vi "Main.vi"(10 "DAQ Type":enum16{"Hardware", "Simulation"}(ring), 11 "Module Admin":refnum<class "Delacor_lib_QMH_Module Admin.lvclass">) -> ()   [LabVIEW 2016, in "CAN.lvlib"]
doc: "This template is based off of the Queued Message Handler design pattern and the Queued Message Handler project template that ships with LabVIEW.\n\nThe main difference is that the queue is private to this module and communication between modules is performed via Broadcast and Request events.\n\nRequest events are wrapped in public API methods and are handled in the Event Handling Loop (EHL) of this VI. Any module can register for Broadcast events sent by this module. The EHL generates messages based on user interface actions.\n\nThe Message Handling Loop (MHL) processes messages generated by the EHL, or by other messages. The messages are string values, so new messages can be added easily to the Message Cases case structure in the MHL. Each message cluster can also provide an optional value for Message Data, which is a variant that can be converted to whatever message-specific data is required.\n_____\nBased on DQMH Project Template 6.1.0.94."
uses:
  CAN.lvlib
  <vilib>/Delacor/Delacor QMH/Libraries/Module Admin_class/Delacor_lib_QMH_Module Admin.lvclass
  Class/Abstract/Abstract.lvclass
  Class/PXI 8513/PXI 8513.lvclass
  D:/common_ATE/Libraries/CAN/Class/Abstract/Abstract.lvclass
  Module Data--cluster.ctl
  <vilib>/Delacor/Delacor QMH/Libraries/Message Queue_class/Delacor_lib_QMH_Message Queue.lvclass/Delacor_lib_QMH_Message Queue.ctl
  Stop Argument--cluster.ctl
  <vilib>/Delacor/Delacor QMH/Libraries/Module Admin_class/Delacor_lib_QMH_Module Admin.lvclass/Delacor_lib_QMH_Module Admin.ctl
  REQ Initialize Hardware Argument--cluster.ctl
  REQ Initialize Hardware (Reply Payload)--cluster.ctl
  REQ Setup Argument--cluster.ctl
  REQ Get Channel Data Argument--cluster.ctl
  REQ CAN Data Argument--cluster.ctl
  REQ Close Ref Argument--cluster.ctl
  <vilib>/Utility/miscctls.llb/LVPointTypeDef.ctl
  <vilib>/Delacor/Delacor QMH/Libraries/Message Queue_class/Delacor_lib_QMH_Enqueue Message (Single).vi
  <vilib>/Delacor/Delacor QMH/Libraries/Module Admin_class/Delacor_lib_QMH_Get External Launch.vi
  <vilib>/Utility/error.llb/Error Cluster From Error Code.vi
  <vilib>/ErrorRing/Error Ring.xnode
  REQ Create CAN Database Argument--cluster.ctl
  <vilib>/Delacor/Delacor QMH/Libraries/Message Queue_class/Delacor_lib_QMH_Message Queue.lvclass
panel:
  out "Session Setting":T1
  out "interface":refnum<k21>
  out "signal list":refnum<k21>[](array[refnum])
  out "Abstract.lvclass":refnum<class "Abstract.lvclass">
  in  "CAN Read?":bool
  out "error out":errorcluster
  out "Status":string
  in  "Simulate MHL Error":bool
  in  "Simulate EHL Error":bool
  # "Other QMH Modules communicate with this Module via its Public API (wrappers for its Request Events).\n\nThis Module communicates with other Modules via its Broadcast Events.\nAny module that wants to get these messages, just registers for this module's Broadcast events."
  # "This template is for the Delacor Modified Queued Message Handler design pattern.\n\nSee the block diagram for more information on how to use this template."
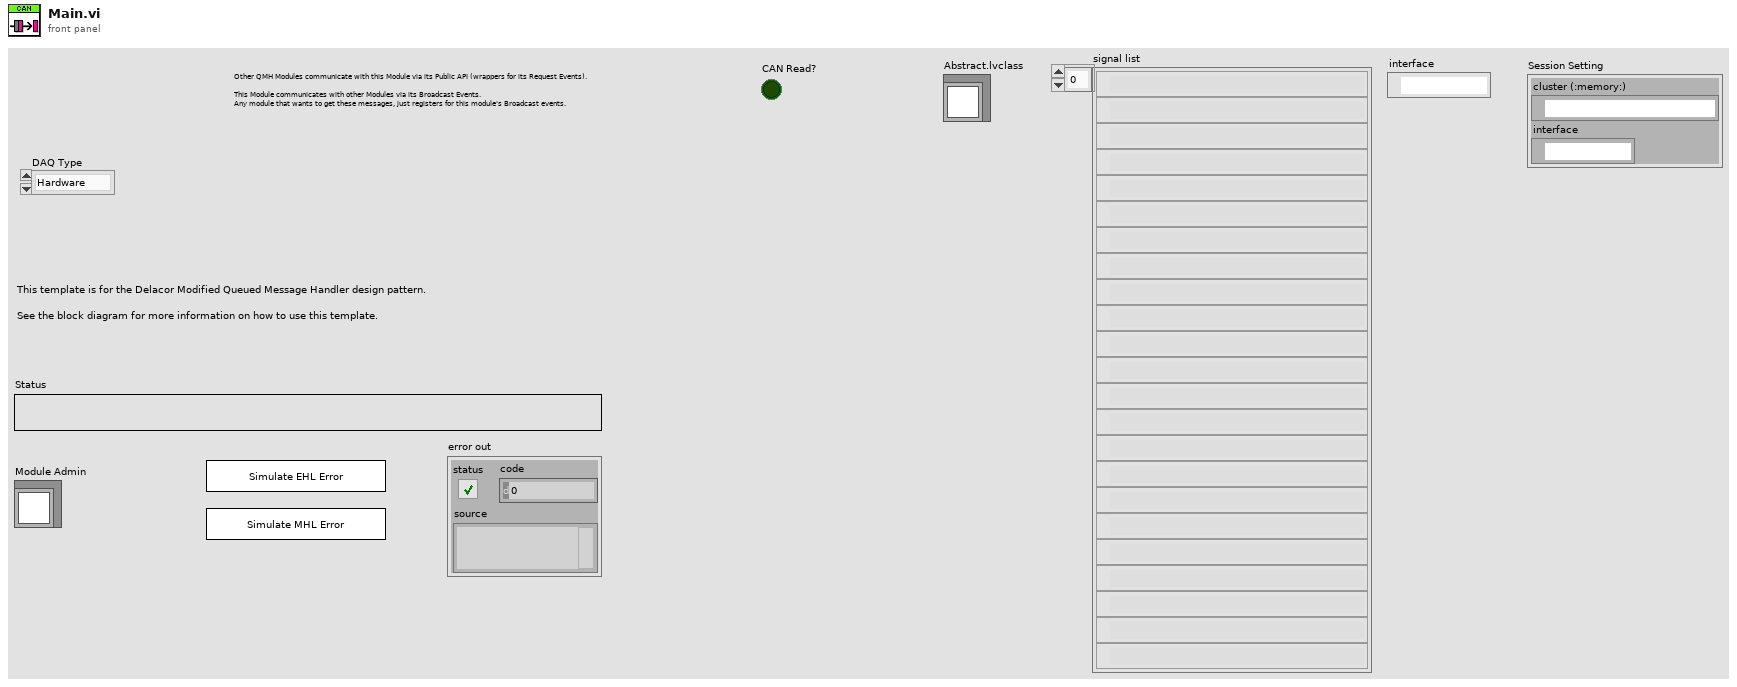
[diagram p1: front panel]
types:
  T1 = cluster{"cluster (:memory:)":refnum<k21>, "interface":refnum<k21>}
  T2 = typedef "CAN.lvlib/Request Events--cluster.ctl" = cluster{"Stop Module":refnum<user-event>, "Show Panel":refnum<user-event>, "Hide Panel":refnum<user-event>, "Get Module Execution Status":refnum<user-event>, "Show Diagram":refnum<user-event>, "REQ Initialize Hardware":refnum<user-event>, "REQ Setup":refnum<user-event>, "REQ Get Channel Data":refnum<user-event>, "REQ CAN Data":refnum<user-event>, "REQ Close Ref":refnum<user-event>, "REQ Create CAN Database":refnum<user-event>}
  T3 = typedef "CAN.lvlib/Module Data--cluster.ctl" = cluster{"Status":string, "Abstract.lvclass":refnum<class "Abstract.lvclass">, "Session Setting":cluster{"cluster (:memory:)":refnum<k21>, "interface":refnum<k21>}, "signal list":refnum<k21>[], "interface":refnum<k21>}
  T4 = enum32{"invalid lock state", "Not Locked", "Locked (No Password)", "Password-protected"}
  T5 = typedef "CAN.lvlib/Stop Argument--cluster.ctl" = cluster{"Origin":string, "Exit via Stop Module Req?":bool, "Wait for Module to stop?":bool}
  T6 = typedef "CAN.lvlib/REQ Initialize Hardware Argument--cluster.ctl" = cluster{"Session Setting":cluster{"cluster (:memory:)":refnum<k21>, "interface":refnum<k21>}, "Connection Ref":variant, "Wait Notifier":refnum<notifier>, "wait for reply":bool}
  T7 = typedef "CAN.lvlib/REQ Setup Argument--cluster.ctl" = cluster{"Setup Setting":cluster{"Interface:64bit Baud Rate":u64, "Interface:CAN:Termination":u32, "Interface:Echo Transmit?":bool}}
  T8 = typedef "CAN.lvlib/REQ Get Channel Data Argument--cluster.ctl" = cluster{"Boolean":bool, "signal list":refnum<k21>[], "interface":refnum<k21>}
  T9 = typedef "CAN.lvlib/REQ CAN Data Argument--cluster.ctl" = cluster{"CAN Read?":bool}
  T10 = typedef "CAN.lvlib/REQ Close Ref Argument--cluster.ctl" = cluster{"Boolean":bool}
  T11 = typedef "CAN.lvlib/REQ Create CAN Database Argument--cluster.ctl" = cluster{"Database Configuration":cluster{"Interface":refnum<k21>, "CAN Cluster":cluster{"Baud Rate":u32, "Comment":string, "Name":string}, "CAN Frame":cluster{"Frame name":string, "Identifier":u32, "Payload Length":u32, "Timing Type":u32, "Transmit Time":dbl, "Extended Identifier?":bool, "Comment":string}, "Signal Cluster":cluster{"Signal name":string, "Scaling Factor":dbl, "Scaling Offset":dbl, "Maximum Value":dbl, "Minimum Value":dbl, "Default Value":dbl, "Unit":string, "Start Bit":u32, "Number of Bits":u32, "Data Type":u32, "Byte Order":u32, "Comment":string}, "Session Type (All Single Point)":enum32{"Signal Input", "Signal Output", "Frame Input", "Frame Output"}}}
  T12 = typedef "LVPointTypeDef.ctl" = cluster{"Horizontal":i16, "Vertical":i16}
  T13 = enum32{"Invalid", "Standard", "Closed", "Hidden", "Minimized", "Maximized"}
  T14 = typedef "CAN.lvlib/REQ Initialize Hardware (Reply Payload)--cluster.ctl" = cluster{"Connect?":bool, "error":errorcluster}
  T15 = cluster{"Interface:64bit Baud Rate":u64, "Interface:CAN:Termination":u32, "Interface:Echo Transmit?":bool}
  T16 = cluster{"Interface":refnum<k21>, "CAN Cluster":cluster{"Baud Rate":u32, "Comment":string, "Name":string}, "CAN Frame":cluster{"Frame name":string, "Identifier":u32, "Payload Length":u32, "Timing Type":u32, "Transmit Time":dbl, "Extended Identifier?":bool, "Comment":string}, "Signal Cluster":cluster{"Signal name":string, "Scaling Factor":dbl, "Scaling Offset":dbl, "Maximum Value":dbl, "Minimum Value":dbl, "Default Value":dbl, "Unit":string, "Start Bit":u32, "Number of Bits":u32, "Data Type":u32, "Byte Order":u32, "Comment":string}, "Session Type (All Single Point)":enum32{"Signal Input", "Signal Output", "Frame Input", "Frame Output"}}
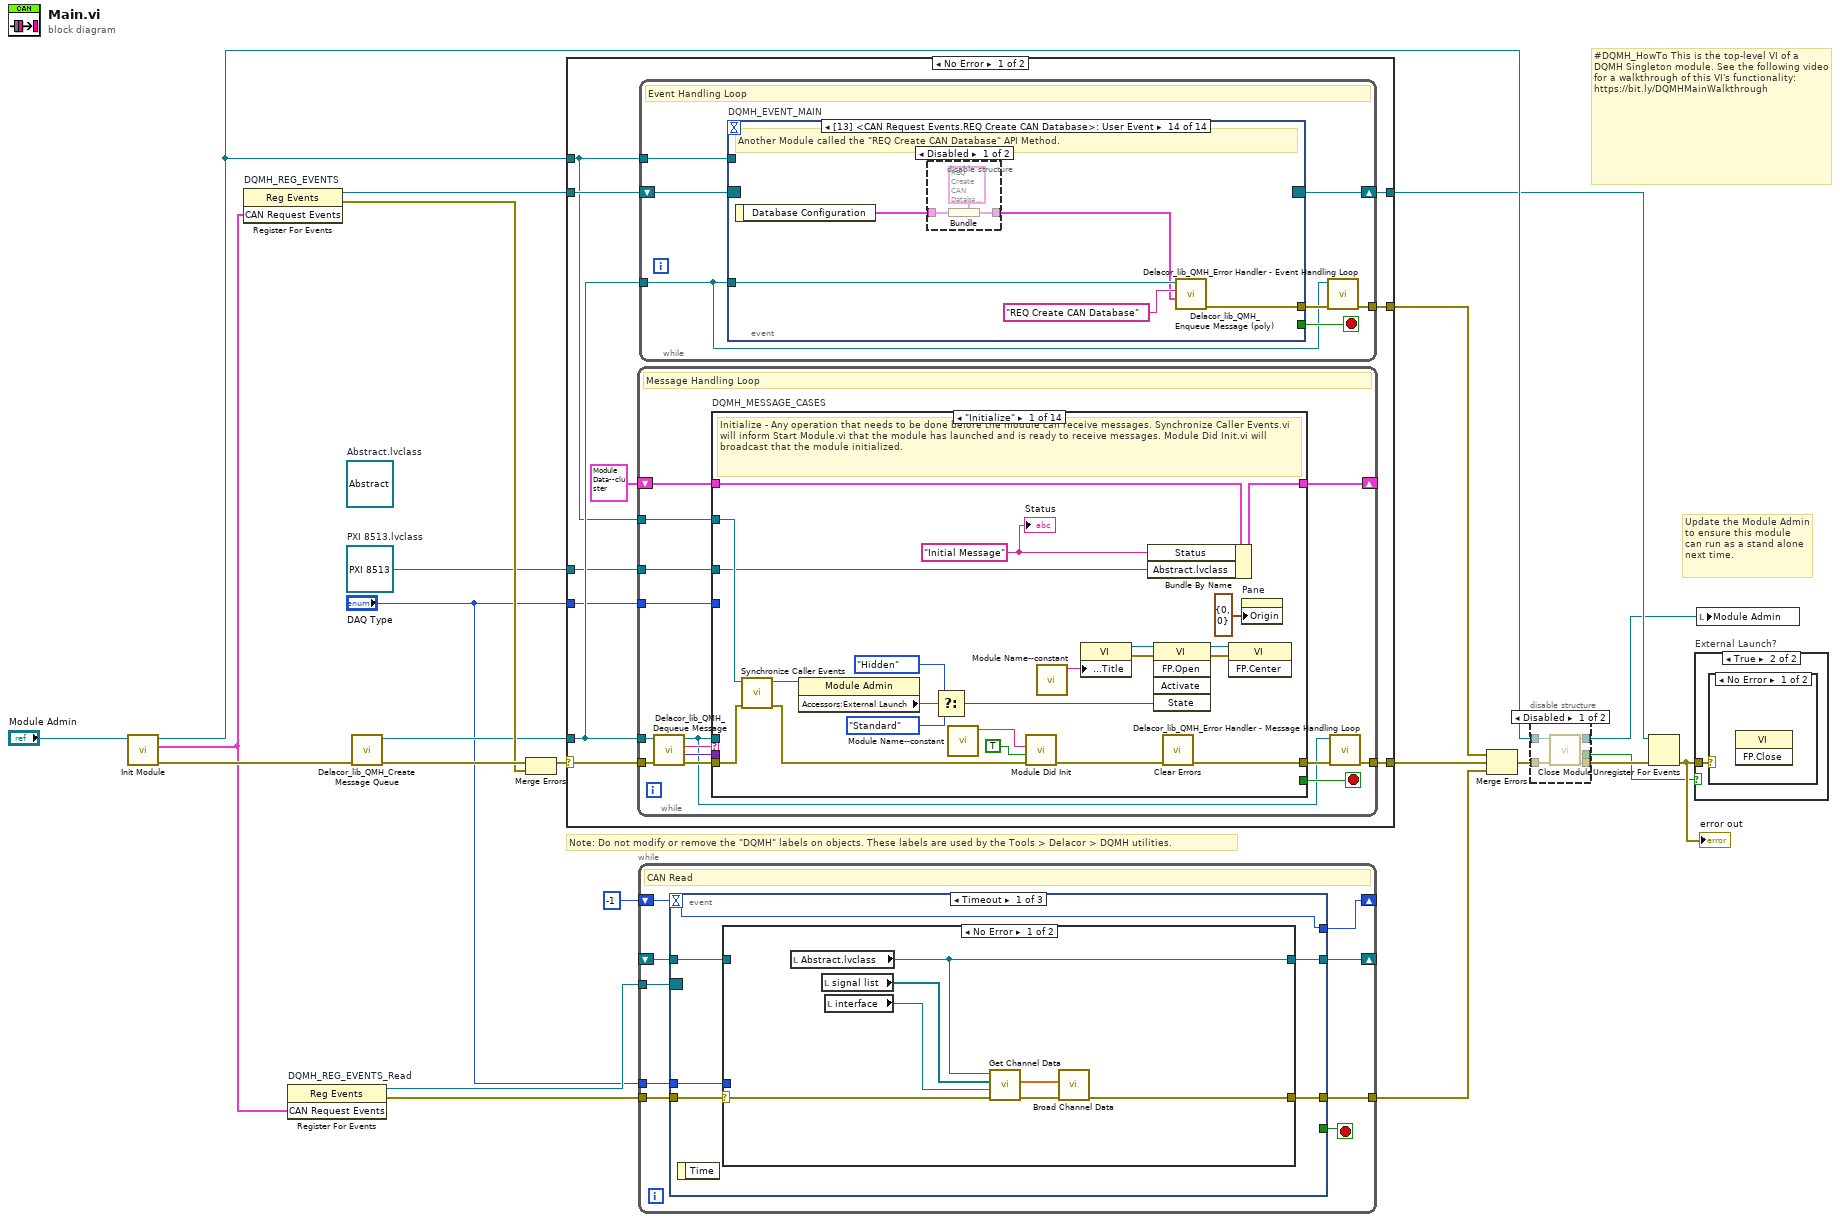
[diagram p0: block diagram]
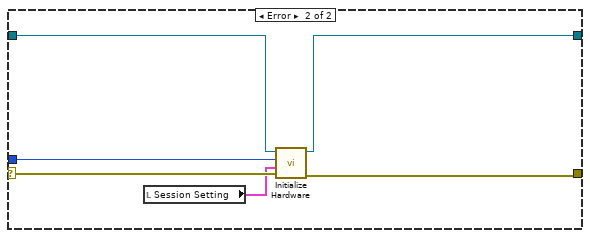
[diagram p3: hidden frame]
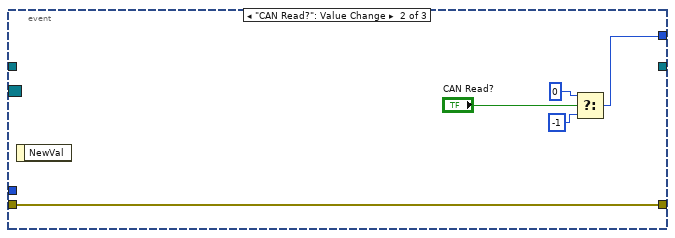
[diagram p4: hidden frame]
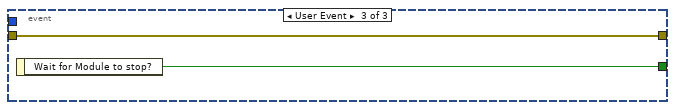
[diagram p5: hidden frame]
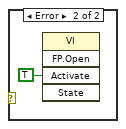
[diagram p7: hidden frame]
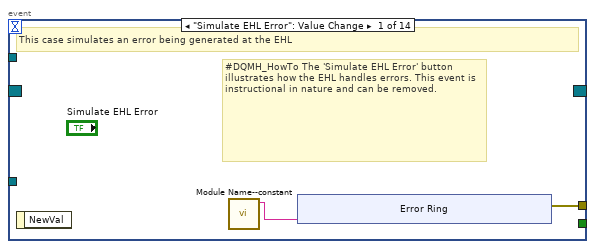
[diagram p8: hidden frame]
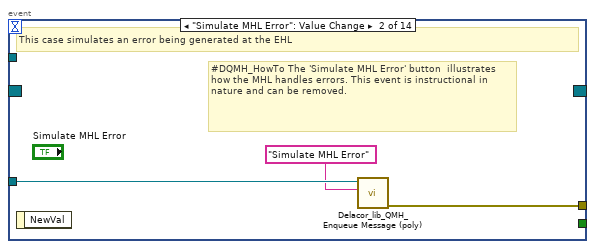
[diagram p9: hidden frame]
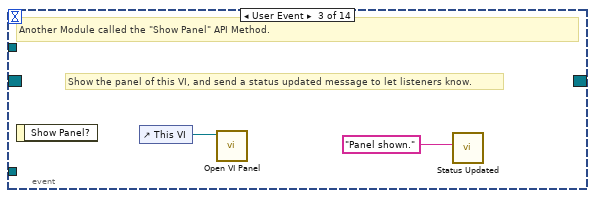
[diagram p10: hidden frame]
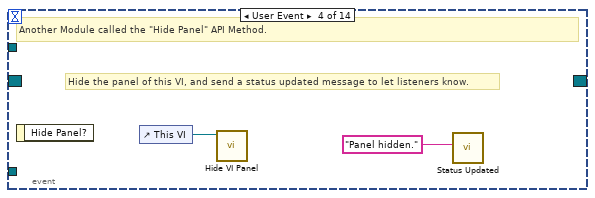
[diagram p11: hidden frame]
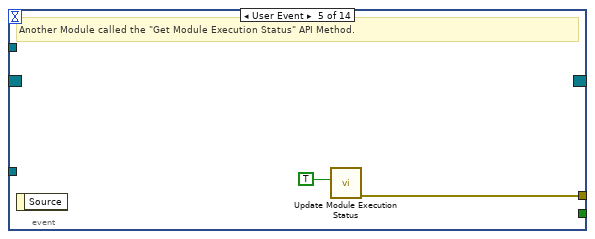
[diagram p12: hidden frame]
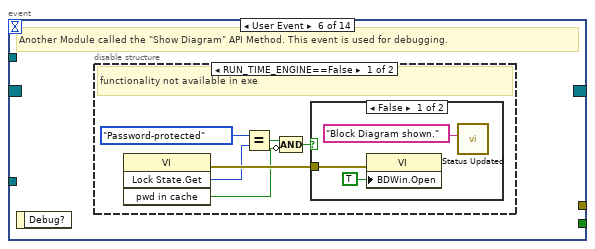
[diagram p13: hidden frame]
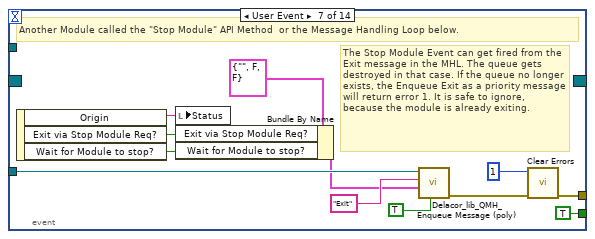
[diagram p16: hidden frame]
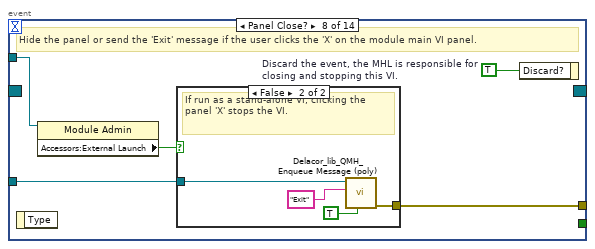
[diagram p17: hidden frame]
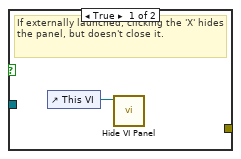
[diagram p18: hidden frame]
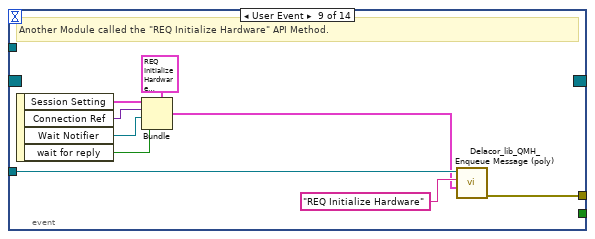
[diagram p19: hidden frame]
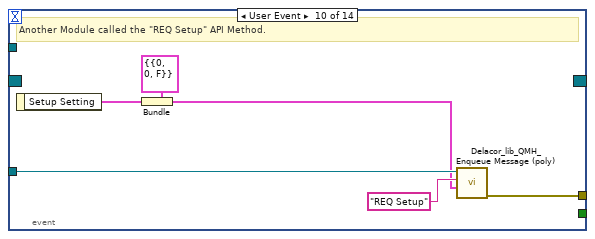
[diagram p20: hidden frame]
diagram:
  w7 = refnum<class "PXI 8513.lvclass"> refnum  # PXI 8513.lvclass
  (unwired) refnum<class "Abstract.lvclass"> refnum  # Abstract.lvclass
  # "#DQMH_HowTo This is the top-level VI of a DQMH Singleton module. See the following video for a walkthrough of this VI's functionality: https://bit.ly/DQMHMainWalkthrough"
  # "Note: Do not modify or remove the \"DQMH\" labels on objects. These labels are used by the Tools > Delacor > DQMH utilities."
  # "Update the Module Admin to ensure this module can run as a stand alone next time."
  n1 = call "Init Module.vi"("Singleton Module Admin in"="Module Admin") -> ("error out"=w22:errorcluster, "CAN Request Events"=w6:T2, "Singleton Module Admin out"=w14:refnum<class "Delacor_lib_QMH_Module Admin.lvclass">)  [unwired: 8 in]
  n2 = register-events "DQMH_REG_EVENTS"(w6) -> (reference out=w12:refnum<event-registration>, error out=w15:errorcluster)  [unwired: 2 in]
  n3 = register-events "DQMH_REG_EVENTS_Read"(w6) -> (reference out=w5:refnum<event-registration>, error out=w4:errorcluster)  [unwired: 2 in]
  n4 = call <vilib>:"Delacor_lib_QMH_Create Message Queue.vi"("error in"=w22) -> ("error out"=w17:errorcluster, "Message Queue"=w11:refnum<class "Delacor_lib_QMH_Message Queue.lvclass">)  [unwired: 9 in]
  n5 = Merge Errors(w17, w15) -> (w16:errorcluster)
  n6 = case shown="No Error" w16 {
    selector: w16 -> [w31 w320]
    tunnel: [w33 w319] -> w23
    tunnel: [w30 w325] -> w13
    tunnel: w12 -> [w28 w325]
    tunnel: w11 -> [w27 w318]
    tunnel: [w32 _] -> w20
    tunnel: w14 -> [w26 w321]
    tunnel: w7 -> [w25 _]
    tunnel: "DAQ Type" -> [w24 _]
    frame No Error {
      n7 = while {
        tunnel: w27 -> [w137]
        shift-right: [w141] -> _
        shift-left: T3 {"Status"="", "Abstract.lvclass"=refnum, "Session Setting"={"cluster (:memory:)"=":memory:", "interface"=""}, "signal list"=[], "interface"=""} ("Data Cluster") -> [w142]
        tunnel: w31 -> [w145]
        tunnel: [w143] -> w33
        tunnel: w26 -> [w135]
        tunnel: w25 -> [w134]
        tunnel: w24 -> [w133]
        stop <- w140 stop-if-true
        # "Message Handling Loop"
        n8 = call-dynamic "Delacor_lib_QMH_Dequeue Message.vi"("error in"=w145, "Message Queue in"=w137) -> ("error out"=w144:errorcluster, "Message Data"=w138:variant, "Message"=w139:string, "Message Queue out"=w136:refnum<class "Delacor_lib_QMH_Message Queue.lvclass">)  [unwired: 6 in]
        n9 = case "DQMH_MESSAGE_CASES" shown="\"Initialize\"" w139 {
          selector: w139 -> [_ _ _ _ _ _ _ _ _ _ _ _ _ w305]
          tunnel: w136 -> [_ _ _ _ _ _ _ _ _ _ _ w271 w293 _]
          tunnel: w144 -> [w166 w170 w189 w202 w211 w223 w229 w239 w254 w256 w261 w278 w299 w307]
          tunnel: [w147 w170 w171 w197 w209 w217 w224 w234 w253 w256 w260 w274 w296 w308] -> w146
          tunnel: w142 -> [w155 w169 w173 w195 w210 w216 w225 w233 w252 w255 w258 w273 w292 w306]
          tunnel: [w154 w169 w180 w193 w205 w216 w225 w231 w252 w255 w258 w273 w292 w306] -> w141
          tunnel: [_ _ _ _ _ _ _ _ _ _ _ _ w291 _] -> w140
          tunnel: w138 -> [_ _ w188 w201 w208 w222 w228 w238 _ _ _ w272 w290 _]
          tunnel: w135 -> [w156 _ _ _ _ _ _ _ _ _ _ w270 w285 _]
          tunnel: w134 -> [w148 _ _ _ _ _ _ _ _ _ _ _ _ _]
          tunnel: w133 -> [_ _ w176 _ _ _ _ _ _ _ _ _ _ _]
          frame "Initialize" {
            w150 = "Initial Message" ("Initial Message")
            # "Initialize - Any operation that needs to be done before the module can receive messages. Synchronize Caller Events.vi will inform Start Module.vi that the module has launched and is ready to receive messages. Module Did Init.vi will broadcast that the module initialized."
            n10 = call "Synchronize Caller Events.vi"("error in (no error)"=w166, "Singleton Module Admin in"=w156) -> ("error out"=w165:errorcluster, "Singleton Module Admin out"=w151:refnum<class "Delacor_lib_QMH_Module Admin.lvclass">)  [unwired: 8 in]
            n11 = property class="Module Admin"(reference=w151) -> ("Accessors:External Launch"=w160:bool)  [unwired: 1 in, 2 out]
            n12 = Select(t=T13."Hidden" ("State"), s=w160, f=T13."Standard" ("State")) -> (s? t:f=w157:T13)
            n13 = call "Module Name--constant.vi"() -> ("Module Name"=w152:string)  [unwired: 11 in]
            n14 = call "Module Did Init.vi"("error in (no error)"=w165, "Initialized?"=TRUE, "Origin"=w152) -> ("error out"=w164:errorcluster)  [unwired: 8 in]
            n15 = call "Module Name--constant.vi"() -> ("Module Name"=w163:string)  [unwired: 11 in]
            n16 = property class="VI"("Front Panel.Title"=w163) -> (reference out=w162:refnum<vi>, error out=w168:errorcluster)  [unwired: 2 in]
            n17 = Bundle By Name(cluster=w155, "Status"=w150, "Abstract.lvclass"=w148) -> (w154:T3)
            n18 = invoke class="VI" method="FP.Open"(reference=w162, error in=w168, "State"=w157) -> (reference out=w161:refnum<vi>, error out=w167:errorcluster)  [unwired: 2 in, 3 out]
            n19 = call <vilib>:"Clear Errors.vi"("error in (no error)"=w164) -> ("error out"=w147:errorcluster)  [unwired: 5 in, 1 out]
            n20 = invoke class="VI" method="FP.Center"(reference=w161, error in=w167) -> ()  [unwired: 1 in, 3 out]
            n21 = property on="Pane" class="Pane"("Origin"=T12 {"Horizontal"=0, "Vertical"=0}) -> ()  [unwired: 2 in, 2 out]
            "Status" <- w150
          }
          frame "---Module Specific---" {
            # "Separator -- The following cases handle messages specific to this Module."
          }
          frame "REQ Initialize Hardware" {
            n22 = Variant To Data(error in=w189, type=T6 {"Session Setting"={"cluster (:memory:)"=":memory:", "interface"=""}, "Connection Ref"=variant, "Wait Notifier"=refnum, "wait for reply"=FALSE} ("REQ Initialize Hardware Argument"), Variant=w188) -> (data=w186:T6, error out=w181:errorcluster)
            n23 = Unbundle By Name(w186) -> ("Wait Notifier"=w185:refnum<notifier>, "wait for reply"=w184:bool, "Session Setting"=w175:T1)
            n24 = Unbundle By Name(w173) -> ("Abstract.lvclass"=w172:refnum<class "Abstract.lvclass">)
            n25 = call-dynamic "Initialize Hardware.vi"("error in (no error)"=w181, "Session Setting"=w175, "DAQ Type"=w176, "Abstract in"=w172) -> ("error out"=w179:errorcluster, "Abstract out"=w174:refnum<class "Abstract.lvclass">)  [unwired: 6 in]
            n26 = Unbundle By Name(w179) -> ("status"=w178:bool)
            n27 = Bundle By Name(cluster=w173, "Session Setting"=w175, "Abstract.lvclass"=w174) -> (w180:T3)
            n28 = Not(x=w178) -> (.not. x?=w177:bool)
            n29 = Bundle By Name(cluster=T14 {"Connect?"=FALSE, "error"={"status"=FALSE, "code"=0, "source"=""}} ("REQ Initialize Hardware (Reply Payload)"), "Connect?"=w177) -> (w183:T14)
            n30 = call <vilib>:"Clear Errors.vi"("error in (no error)"=w179) -> ("error out"=w171:errorcluster)  [unwired: 5 in, 1 out]
            n31 = case shown="True" w184 {
              tunnel: w185 -> [_ w191]
              tunnel: w183 -> [_ w190]
              frame False {
              }
              frame True {
                n32 = Send Notification(notification=w190, notifier=w191) -> ()  [unwired: 1 in, 2 out]
              }
            }
          }
          frame "REQ Setup" {
            n33 = Variant To Data(error in=w202, type=T7 {"Setup Setting"={"Interface:64bit Baud Rate"=0, "Interface:CAN:Termination"=0, "Interface:Echo Transmit?"=FALSE}} ("REQ Setup Argument"), Variant=w201) -> (data=w199:T7, error out=w198:errorcluster)
            n34 = Unbundle By Name(w199) -> ("Setup Setting"=w196:T15)
            n35 = Unbundle By Name(w195) -> ("Abstract.lvclass"=w194:refnum<class "Abstract.lvclass">)
            n36 = call-dynamic "Setup.vi"("error in (no error)"=w198, "Setup Setting"=w196, "Abstract in"=w194) -> ("error out"=w197:errorcluster, "Abstract out"=w192:refnum<class "Abstract.lvclass">)  [unwired: 7 in]
            n37 = Bundle By Name(cluster=w195, "Abstract.lvclass"=w192) -> (w193:T3)
          }
          frame "REQ Get Channel Data" {
            n38 = Variant To Data(error in=w211, type=T8 {"Boolean"=FALSE, "signal list"=[], "interface"=""} ("REQ Get Channel Data Argument"), Variant=w208) -> (data=w206:T8, error out=w209:errorcluster)
            n39 = Unbundle By Name(w206) -> ("signal list"=w204:refnum<k21>[], "interface"=w203:refnum<k21>)
            n40 = Bundle By Name(cluster=w210, "signal list"=w204, "interface"=w203) -> (w205:T3)
          }
          frame "REQ CAN Data" {
            n41 = Variant To Data(error in=w223, type=T9 {"CAN Read?"=FALSE} ("REQ CAN Data Argument"), Variant=w222) -> (data=w220:T9, error out=w218:errorcluster)
            n42 = Unbundle By Name(w220) -> ("CAN Read?"=w219:bool)
            n43 = Unbundle By Name(w216) -> ("Abstract.lvclass"=→"Abstract.lvclass":refnum<class "Abstract.lvclass">, "signal list"=→"signal list":refnum<k21>[], "interface"=→"interface":refnum<k21>, "Session Setting"=→"Session Setting":T1)
            n44 = property on="CAN Read?" class="Bool (strict)"(error in=w218, "Val(Sgnl)"=w219) -> (error out=w217:errorcluster)  [unwired: 1 in, 1 out]
          }
          frame "REQ Close Ref" {
            n45 = Variant To Data(error in=w229, type=T10 {"Boolean"=FALSE} ("REQ Close Ref Argument"), Variant=w228) -> (data=w226:T10, error out=w224:errorcluster)
            n46 = Unbundle By Name(w226) -> ()  [unwired: 1 out]
            n47 = Unbundle By Name(w225) -> ()  [unwired: 1 out]
          }
          frame "REQ Create CAN Database" {
            n48 = disable-structure shown="Enabled" {
              disable-tunnel: w239 -> [w244 w245]
              disable-tunnel: w238 -> [w243 _]
              disable-tunnel: [w241 _] -> w237
              disable-tunnel: [w240 w245] -> w236
              frame Disabled {
                n49 = Variant To Data(error in=w244, type=T11 {"Database Configuration"={"Interface"="CAN1", "CAN Cluster"={"Baud Rate"=125000, "Comment"="", "Name"="CAN_Cluster"}, "CAN Frame"={"Frame name"="frame1", "Identifier"=1, "Payload Length"=8, "Timing Type"=1, "Transmit Time"=0.0, "Extended Identifier?"=FALSE, "Comment"=""}, "Signal Cluster"={"Signal name"="signal", "Scaling Factor"=1.0, "Scaling Offset"=0.0, "Maximum Value"=256.0, "Minimum Value"=0.0, "Default Value"=0.0, "Unit"="V", "Start Bit"=0, "Number of Bits"=8, "Data Type"=1, "Byte Order"=0, "Comment"=""}, "Session Type (All Single Point)"=enum."Signal Input"}} ("REQ Create CAN Database Argument"), Variant=w243) -> (data=w241:T11, error out=w240:errorcluster)
              }
              frame Enabled {
              }
            }
            n50 = Unbundle By Name(w237) -> ("Database Configuration"=w235:T16)
            n51 = Unbundle By Name(w233) -> ("Abstract.lvclass"=w232:refnum<class "Abstract.lvclass">)
            n52 = disable-structure shown="Enabled" {
              disable-tunnel: w236 -> [w250 w251]
              disable-tunnel: w235 -> [w249 _]
              disable-tunnel: [w248 w251] -> w234
              disable-tunnel: w232 -> [w247 _]
              disable-tunnel: [w246 _] -> w230
              frame Disabled {
                n53 = call-dynamic "Create Database.vi"("error in (no error)"=w250, "Database Configuration"=w249, "Abstract in"=w247) -> ("error out"=w248:errorcluster, "Abstract out"=w246:refnum<class "Abstract.lvclass">)  [unwired: 7 in]
              }
              frame Enabled {
              }
            }
            n54 = Bundle By Name(cluster=w233, "Abstract.lvclass"=w230) -> (w231:T3)
          }
          frame "---Copy This Frame---" {
            # "Duplicate this frame when creating new messages.  Change this comment in the duplicated frame to describe this message."
            n55 = Merge Errors(w254) -> (w253:errorcluster)
          }
          frame "---Exit and Error Handling---" {
            # "Separator - The following cases handle errors and exit messages."
          }
          frame "Simulate MHL Error" {
            # "#DQMH_HowTo The 'Simulate MHL Error' button  illustrates how the MHL handles errors. This event is instructional in nature and can be removed."
            # "Simulate an error occurring at the MHL"
            n56 = call "Module Name--constant.vi"() -> ("Module Name"=w257:string)  [unwired: 11 in]
            n57 = xnode "Error Ring"("parameter 0"=w257) -> ("error out"=w259:errorcluster)
            n58 = Merge Errors(w261, w259) -> (w260:errorcluster)
          }
          frame "Error" {
            # "#CodeRecommended - If you ever change the name of this \"Error\" message, you'll need to update the name in the Check Loop Error.vi as well."
            # "#CodeRecommended - If the module is running in standalone mode (External Launch = FALSE), this code will pop up an error dialog and call the 'Exit' message if an error occurs. Add more fine-grained error handling here."
            # "Error - Check the error message data and respond accordingly. This message is sent by the \"Error Handler\" VIs at the end of each loop in this application."
            n59 = property class="Module Admin"(reference=w270) -> ("Accessors:External Launch"=w269:bool)  [unwired: 1 in, 2 out]
            n60 = Variant To Data(error in=w278, type=errorcluster {"status"=FALSE, "code"=0, "source"=""} ("error constant"), Variant=w272) -> (data=w279:errorcluster, error out=w276:errorcluster)
            n61 = call "Error Reported.vi"("Error"=w279) -> ()  [unwired: 10 in, 1 out]
            n62 = case shown="False" w269 {
              tunnel: [w284 _] -> w275
              tunnel: w271 -> [w282 _]
              tunnel: w279 -> [w283 _]
              frame False {
                # "If the module is running standalone, then pop up an error dialog and call the \"Exit\" message."
                n63 = call <vilib>:"Simple Error Handler.vi"("error in (no error)"=w283) -> ()  [unwired: 4 in, 5 out]
                n64 = call-poly <vilib>:"Delacor_lib_QMH_Enqueue Message (poly).vi"("Priority Message? (F)"=TRUE, "Message"="Exit", "Message Queue in"=w282) -> ("error out"=w284:errorcluster)  [unwired: 7 in, 1 out]
              }
              frame True {
                # "If the module was launched externally, calling the Error Reported broadcast VI is the only action performed by the \"Error\" message. The module's caller can then process the error appropriately."
              }
            }
            n65 = Merge Errors(w276, w275) -> (w274:errorcluster)
            n66 = local write "error out"(w274) -> ()
          }
          frame "Exit" {
            w289 = 91  # 91: not all Exit messages will have an argument
            w291 = TRUE  # Stop the VI
            # "Release the message queue reference"
            # "#CodeNeeded - Add any required cleanup code here"
            # "Exit - Exit the application."
            n67 = Variant To Data(error in=w299, type=T5 {"Origin"="", "Exit via Stop Module Req?"=FALSE, "Wait for Module to stop?"=FALSE} ("Stop Argument"), Variant=w290) -> (data=w287:T5, error out=w295:errorcluster)
            n68 = call <vilib>:"Clear Errors.vi"("error in (no error)"=w295, "specific error code to clear (0: all)"=w289) -> ("error out"=w298:errorcluster)  [unwired: 4 in, 1 out]
            n69 = control-ref of="This VI"() -> (w286:refnum<vi>)
            n70 = disable-structure shown="Disabled" {
              disable-tunnel: [w303 _] -> w294
              disable-tunnel: w287 -> [w302 _]
              disable-tunnel: w286 -> [w301 _]
              disable-tunnel: w285 -> [w300 _]
              frame Disabled {
                n71 = call "Handle Exit.vi"("Stop Argument"=w302, "Admin in"=w300, "VI reference"=w301) -> ("error out"=w303:errorcluster)  [unwired: 7 in, 1 out]
              }
              frame Enabled {
              }
            }
            n72 = call-dynamic "Delacor_lib_QMH_Release Message Queue.vi"("error in"=w298, "Message Queue"=w293) -> ("error out"=w297:errorcluster)  [unwired: 9 in]
            n73 = Merge Errors(w297, w294) -> (w296:errorcluster)
          }
          frame Default {
            # "'Default' case only runs if there is a message that isn't defined in any of the other cases.  Output a programming error."
            n74 = call "Module Name--constant.vi"() -> ("Module Name"=w304:string)  [unwired: 11 in]
            n75 = xnode "Error Ring"("parameter 0"=w305, "parameter 1"=w304) -> ("error out"=w309:errorcluster)
            n76 = Merge Errors(w307, w309) -> (w308:errorcluster)
          }
        }
        n77 = call-dynamic "Delacor_lib_QMH_Error Handler - Message Handling Loop.vi"("error in"=w146, "Message Queue in"=w136) -> ("dup error in"=w143:errorcluster)  [unwired: 8 in, 1 out]
      }
      n78 = while {
        tunnel: w27 -> [w34]
        shift-right: [w37] -> w30
        shift-left: w28 -> [w38]
        tunnel: [w39] -> w32
        tunnel: w26 -> [w35]
        stop <- w36 stop-if-true
        # "Event Handling Loop"
        n79 = event "DQMH_EVENT_MAIN" shown="[13] <CAN Request Events.REQ Create CAN Database>: User Event" {
          selector: w38 -> [_ _ _ _ _ _ _ _ _ _ _ _ _ _]
          dyn-events: [_ _ _ _ _ _ _ _ _ _ _ _ _ _] -> w37
          timeout: _ -> [_ _ _ _ _ _ _ _ _ _ _ _ _ _]
          tunnel: [_ _ _ _ _ _ TRUE ("Discard?") _ _ _ _ _ _ _] -> w36
          tunnel: w34 -> [_ w51 _ _ _ _ w75 w82 w98 w104 w112 w118 w124 w129]
          tunnel: [w42 w52 _ _ w58 _ w78 w84 w90 w99 w107 w113 w119 w125] -> w40
          tunnel: w35 -> [_ _ _ _ _ _ _ w81 _ _ _ _ _ _]
          event "Simulate EHL Error": Value Change {
            # "#DQMH_HowTo The 'Simulate EHL Error' button  illustrates how the EHL handles errors. This event is instructional in nature and can be removed."
            # "This case simulates an error being generated at the EHL"
            n80 = event-data() -> ()  [unwired: 1 in, 1 out]
            n81 = call "Module Name--constant.vi"() -> ("Module Name"=w41:string)  [unwired: 11 in]
            n82 = xnode "Error Ring"("parameter 0"=w41) -> ("error out"=w42:errorcluster)
          }
          event "Simulate MHL Error": Value Change {
            # "#DQMH_HowTo The 'Simulate MHL Error' button  illustrates how the MHL handles errors. This event is instructional in nature and can be removed."
            # "This case simulates an error being generated at the EHL"
            n83 = event-data() -> ()  [unwired: 1 in, 1 out]
            n84 = call-poly <vilib>:"Delacor_lib_QMH_Enqueue Message (poly).vi"("Message"="Simulate MHL Error", "Message Queue in"=w51) -> ("error out"=w52:errorcluster)  [unwired: 8 in, 1 out]
          }
          event User Event {
            # "Show the panel of this VI, and send a status updated message to let listeners know."
            # "Another Module called the \"Show Panel\" API Method."
            n85 = event-data() -> ()  [unwired: 1 in, 1 out]
            n86 = control-ref of="This VI"() -> (w54:refnum<vi>)
            n87 = call "Open VI Panel.vi"("VI"=w54) -> ()  [unwired: 10 in, 1 out]
            n88 = call "Status Updated.vi"("Status"="Panel shown." ("format string")) -> ()  [unwired: 10 in, 1 out]
          }
          event User Event {
            # "Hide the panel of this VI, and send a status updated message to let listeners know."
            # "Another Module called the \"Hide Panel\" API Method."
            n89 = event-data() -> ()  [unwired: 1 in, 1 out]
            n90 = control-ref of="This VI"() -> (w56:refnum<vi>)
            n91 = call "Hide VI Panel.vi"("VI"=w56) -> ()  [unwired: 10 in, 1 out]
            n92 = call "Status Updated.vi"("Status"="Panel hidden." ("format string")) -> ()  [unwired: 10 in, 1 out]
          }
          event User Event {
            # "Another Module called the \"Get Module Execution Status\" API Method."
            n93 = event-data() -> ()  [unwired: 1 in, 1 out]
            n94 = call "Update Module Execution Status.vi"("Running?"=TRUE) -> ("error out"=w58:errorcluster)  [unwired: 10 in]
          }
          event User Event {
            # "Another Module called the \"Show Diagram\" API Method. This event is used for debugging."
            n95 = event-data() -> ()  [unwired: 1 in, 1 out]
            n96 = disable-structure shown="RUN_TIME_ENGINE==False" {
              frame condition #0 (active) {
                # "functionality not available in exe"
                n97 = invoke class="VI" method="Lock State.Get"() -> (error out=w64:errorcluster, "Get Lock State"=w63:T4, "pwd in cache"=w60:bool)  [unwired: 4 in, 1 out]
                n98 = Equal?(x=T4."Password-protected", y=w63) -> (x = y?=w61:bool)
                n99 = Compound Arithmetic op=AND(w61, invert w60) -> (w59:bool)
                n100 = case shown="False" w59 {
                  tunnel: w64 -> [w67 _]
                  frame False {
                    n101 = property class="VI"(error in=w67, "BDWin.Open"=TRUE ("Block Diagram Window:Open")) -> ()  [unwired: 1 in, 2 out]
                    n102 = call "Status Updated.vi"("Status"="Block Diagram shown." ("format string")) -> ()  [unwired: 10 in, 1 out]
                  }
                  frame True {
                    # "Password-protected VI, and the password is not in the cache. Do not show the diagram."
                  }
                }
              }
              frame condition #1 {
              }
            }
          }
          event User Event {
            # "The Stop Module Event can get fired from the Exit message in the MHL. The queue gets destroyed in that case. If the queue no longer exists, the Enqueue Exit as a priority message will return error 1. It is safe to ignore, because the module is already exiting."
            # "Another Module called the \"Stop Module\" API Method  or the Message Handling Loop below."
            n103 = event-data() -> ("Origin"=w74:string, "Exit via Stop Module Req?"=w70:bool, "Wait for Module to stop?"=w69:bool)  [unwired: 1 in]
            n104 = local write "Status"(w74) -> ()
            n105 = Bundle By Name(cluster=T5 {"Origin"="", "Exit via Stop Module Req?"=FALSE, "Wait for Module to stop?"=FALSE} ("Stop Argument"), "Exit via Stop Module Req?"=w70, "Wait for Module to stop?"=w69) -> (w68:T5)
            n106 = call-poly <vilib>:"Delacor_lib_QMH_Enqueue Message (poly).vi"("Priority Message? (F)"=TRUE, "Message Data"=w68, "Message"="Exit", "Message Queue in"=w75) -> ("error out"=w79:errorcluster)  [unwired: 6 in, 1 out]
            n107 = call <vilib>:"Clear Errors.vi"("error in (no error)"=w79, "specific error code to clear (0: all)"=1) -> ("error out"=w78:errorcluster)  [unwired: 4 in, 1 out]
          }
          event Panel Close? {
            w83 = TRUE  # Discard the event, the MHL is responsible for closing and stopping this VI.
            # "Hide the panel or send the 'Exit' message if the user clicks the 'X' on the module main VI panel."
            n108 = event-data() -> ()  [unwired: 1 in, 1 out]
            n109 = property class="Module Admin"(reference=w81) -> ("Accessors:External Launch"=w80:bool)  [unwired: 1 in, 2 out]
            n110 = case shown="False" w80 {
              tunnel: w82 -> [_ w88]
              tunnel: [_ w89] -> w84
              frame True {
                # "If externally launched, clicking the 'X' hides the panel, but doesn't close it."
                n111 = control-ref of="This VI"() -> (w85:refnum<vi>)
                n112 = call "Hide VI Panel.vi"("VI"=w85) -> ()  [unwired: 10 in, 1 out]
              }
              frame False {
                # "If run as a stand-alone VI, clicking the panel 'X' stops the VI."
                n113 = call-poly <vilib>:"Delacor_lib_QMH_Enqueue Message (poly).vi"("Priority Message? (F)"=TRUE, "Message"="Exit", "Message Queue in"=w88) -> ("error out"=w89:errorcluster)  [unwired: 7 in, 1 out]
              }
            }
            n114 = event-data("Discard?"=w83) -> ()  [unwired: 1 in, 1 out]
          }
          event User Event {
            # "Another Module called the \"REQ Initialize Hardware\" API Method."
            n115 = event-data() -> ("Session Setting"=w94:T1, "Connection Ref"=w93:variant, "Wait Notifier"=w92:refnum<notifier>, "wait for reply"=w91:bool)  [unwired: 1 in]
            n116 = Bundle(cluster=T6 {"Session Setting"={"cluster (:memory:)"=":memory:", "interface"=""}, "Connection Ref"=variant, "Wait Notifier"=refnum, "wait for reply"=FALSE} ("REQ Initialize Hardware Argument"), "Session Setting"=w94, "Connection Ref"=w93, "Wait Notifier"=w92, "wait for reply"=w91) -> (w95:T6)
            n117 = call-poly <vilib>:"Delacor_lib_QMH_Enqueue Message (poly).vi"("Message Data"=w95, "Message"="REQ Initialize Hardware", "Message Queue in"=w98) -> ("error out"=w90:errorcluster)  [unwired: 7 in, 1 out]
          }
          event User Event {
            # "Another Module called the \"REQ Setup\" API Method."
            n118 = event-data() -> ("Setup Setting"=w100:T15)  [unwired: 1 in]
            n119 = Bundle(cluster=T7 {"Setup Setting"={"Interface:64bit Baud Rate"=0, "Interface:CAN:Termination"=0, "Interface:Echo Transmit?"=FALSE}} ("REQ Setup Argument"), "Setup Setting"=w100) -> (w101:T7)
            n120 = call-poly <vilib>:"Delacor_lib_QMH_Enqueue Message (poly).vi"("Message Data"=w101, "Message"="REQ Setup", "Message Queue in"=w104) -> ("error out"=w99:errorcluster)  [unwired: 7 in, 1 out]
          }
          event User Event {
            # "Another Module called the \"REQ Get Channel Data\" API Method."
            n121 = event-data() -> ("Boolean"=w108:bool, "signal list"=w106:refnum<k21>[], "interface"=w105:refnum<k21>)  [unwired: 1 in]
            n122 = Bundle(cluster=T8 {"Boolean"=FALSE, "signal list"=[], "interface"=""} ("REQ Get Channel Data Argument"), "Boolean"=w108, "signal list"=w106, "interface"=w105) -> (w109:T8)
            n123 = call-poly <vilib>:"Delacor_lib_QMH_Enqueue Message (poly).vi"("Message Data"=w109, "Message"="REQ Get Channel Data", "Message Queue in"=w112) -> ("error out"=w107:errorcluster)  [unwired: 7 in, 1 out]
          }
          event User Event {
            # "Another Module called the \"REQ CAN Data\" API Method."
            n124 = event-data() -> ("CAN Read?"=w114:bool)  [unwired: 1 in]
            n125 = Bundle(cluster=T9 {"CAN Read?"=FALSE} ("REQ CAN Data Argument"), "CAN Read?"=w114) -> (w115:T9)
            n126 = call-poly <vilib>:"Delacor_lib_QMH_Enqueue Message (poly).vi"("Message Data"=w115, "Message"="REQ CAN Data", "Message Queue in"=w118) -> ("error out"=w113:errorcluster)  [unwired: 7 in, 1 out]
          }
          event User Event {
            # "Another Module called the \"REQ Close Ref\" API Method."
            n127 = event-data() -> ("Boolean"=w120:bool)  [unwired: 1 in]
            n128 = Bundle(cluster=T10 {"Boolean"=FALSE} ("REQ Close Ref Argument"), "Boolean"=w120) -> (w121:T10)
            n129 = call-poly <vilib>:"Delacor_lib_QMH_Enqueue Message (poly).vi"("Message Data"=w121, "Message"="REQ Close Ref", "Message Queue in"=w124) -> ("error out"=w119:errorcluster)  [unwired: 7 in, 1 out]
          }
          event User Event {
            # "Another Module called the \"REQ Create CAN Database\" API Method."
            n130 = event-data() -> ("Database Configuration"=w126:T16)  [unwired: 1 in]
            n131 = disable-structure shown="Disabled" {
              disable-tunnel: [w131 _] -> w127
              disable-tunnel: w126 -> [w130 _]
              frame Disabled {
                n132 = Bundle(cluster=T11 {"Database Configuration"={"Interface"="CAN1", "CAN Cluster"={"Baud Rate"=125000, "Comment"="", "Name"="CAN_Cluster"}, "CAN Frame"={"Frame name"="frame1", "Identifier"=1, "Payload Length"=8, "Timing Type"=1, "Transmit Time"=0.0, "Extended Identifier?"=FALSE, "Comment"=""}, "Signal Cluster"={"Signal name"="signal", "Scaling Factor"=1.0, "Scaling Offset"=0.0, "Maximum Value"=256.0, "Minimum Value"=0.0, "Default Value"=0.0, "Unit"="V", "Start Bit"=0, "Number of Bits"=8, "Data Type"=1, "Byte Order"=0, "Comment"=""}, "Session Type (All Single Point)"=enum."Signal Input"}} ("REQ Create CAN Database Argument"), "Database Configuration"=w130) -> (w131:T11)
              }
              frame Enabled {
              }
            }
            n133 = call-poly <vilib>:"Delacor_lib_QMH_Enqueue Message (poly).vi"("Message Data"=w127, "Message"="REQ Create CAN Database", "Message Queue in"=w129) -> ("error out"=w125:errorcluster)  [unwired: 7 in, 1 out]
          }
        }
        n134 = call-dynamic "Delacor_lib_QMH_Error Handler - Event Handling Loop.vi"("error in"=w40, "Message Queue in"=w34) -> ("dup error in"=w39:errorcluster)  [unwired: 8 in, 1 out]
      }
    }
    frame Error {
      # "Synchronize Caller Events.vi will inform Start Module.vi that the module has launched and will let the code calling Start Module.vi register for broadcasts and would permit the caller receive the broadcast that an error occurred at launch time."
      n135 = call-dynamic "Delacor_lib_QMH_Release Message Queue.vi"("error in"=w320, "Message Queue"=w318) -> ("error out"=w319:errorcluster)  [unwired: 9 in]
      n136 = call "Synchronize Caller Events.vi"("Singleton Module Admin in"=w321) -> ("error out"=w326:errorcluster)  [unwired: 9 in, 1 out]
      n137 = call "Module Name--constant.vi"() -> ("Module Name"=w324:string)  [unwired: 11 in]
      n138 = Format Into String(format string="An error occurred during initialization. %s is no longer running.", w324) -> (resulting string=w322:string)  [unwired: 2 in, 1 out]
      n139 = Merge Errors(w319, w326) -> (w327:errorcluster)
      n140 = call "Error Reported.vi"("Additional Information"=w322, "Error"=w327) -> ()  [unwired: 9 in, 1 out]
    }
  }
  n141 = while {
    tunnel: w5 -> [w336]
    tunnel: w4 -> [w335]
    tunnel: [w333] -> w3
    shift-right: [w331] -> _
    shift-left: -1 -> [w332]
    shift-right: [w330] -> _
    shift-left: _ -> [w329]
    tunnel: "DAQ Type" -> [w328]
    stop <- w334 stop-if-true
    # "CAN Read"
    n142 = event shown="[0] Timeout" {
      selector: w336 -> [_ _ _]
      dyn-events: _ -> [_ _ _]
      timeout: w332 -> [w342 _ _]
      tunnel: w335 -> [w341 w356 w361]
      tunnel: [_ _ w362] -> w334
      tunnel: [w340 w356 w361] -> w333
      tunnel: [w342 w357 _] -> w331
      tunnel: [w339 _ _] -> w330
      tunnel: w329 -> [w338 _ _]
      tunnel: w328 -> [w337 _ _]
      event Timeout {
        n143 = event-data() -> ()  [unwired: 1 in, 1 out]
        n144 = case shown="No Error" w341 {
          selector: w341 -> [w349 w354]
          tunnel: [w344 w353] -> w340
          tunnel: [w346 w352] -> w339
          tunnel: w338 -> [_ w355]
          tunnel: w337 -> [_ w351]
          frame No Error {
            n145 = local read "Abstract.lvclass"() -> (w346:refnum<class "Abstract.lvclass">)
            n146 = local read "signal list"() -> (w348:refnum<k21>[])
            n147 = local read "interface"() -> (w347:refnum<k21>)
            n148 = call-dynamic "Get Channel Data.vi"("error in (no error)"=w349, "interface"=w347, "signal list"=w348, "Abstract in"=w346) -> ("error out"=w345:errorcluster, "Data"=w343:dbl[])  [unwired: 5 in, 1 out]
            n149 = call "Broad Channel Data.vi"("error in"=w345, "Data"=w343) -> ("error out"=w344:errorcluster)  [unwired: 9 in]
          }
          frame Error {
            n150 = local read "Session Setting"() -> (w350:T1)
            n151 = call-dynamic "Initialize Hardware.vi"("error in (no error)"=w354, "Session Setting"=w350, "DAQ Type"=w351, "Abstract in"=w355) -> ("error out"=w353:errorcluster, "Abstract out"=w352:refnum<class "Abstract.lvclass">)  [unwired: 6 in]
          }
        }
      }
      event "CAN Read?": Value Change {
        n152 = event-data() -> ()  [unwired: 1 in, 1 out]
        n153 = Select(t=0, s="CAN Read?", f=-1) -> (s? t:f=w357:i32)
      }
      event User Event {
        n154 = event-data() -> ("Wait for Module to stop?"=w362:bool)  [unwired: 1 in]
      }
    }
  }
  n155 = Merge Errors(w20, w23, w3) -> (w19:errorcluster)
  n156 = disable-structure shown="Disabled" {
    disable-tunnel: [w367 _] -> w21
    disable-tunnel: w19 -> [w366 _]
    disable-tunnel: w14 -> [w365 _]
    disable-tunnel: [w364 _] -> w9
    disable-tunnel: [w363 _] -> w8
    frame Disabled {
      n157 = call "Close Module.vi"("error in (no error)"=w366, "Module Admin in"=w365) -> ("error out"=w367:errorcluster, "External Launch"=w363:bool, "Module Admin out"=w364:refnum<class "Delacor_lib_QMH_Module Admin.lvclass">)  [unwired: 7 in]
    }
    frame Enabled {
    }
  }
  n158 = Unregister For Events(event registration refnum=w13, error in=w21) -> (error out=w18:errorcluster)
  "error out" <- w18
  n159 = case "External Launch?" shown="True" w8 {
    tunnel: w18 -> [_ w368]
    frame False {
    }
    frame True {
      n160 = case shown="No Error" w368 {
        frame No Error {
          n161 = invoke class="VI" method="FP.Close"() -> ()  [unwired: 3 in, 3 out]
        }
        frame Error {
          n162 = invoke class="VI" method="FP.Open"("Activate"=TRUE ("Activate?")) -> ()  [unwired: 4 in, 5 out]
        }
      }
    }
  }
  n163 = local write "Module Admin"(w9) -> ()
